vi "AOI_Main.vi"() -> ()   [LabVIEW 2017]
uses:
  <vilib>/userdefined/High Color/IMAQdx.ctl
  <vilib>/vision/driver/IMAQdx.llb/IMAQdx Camera Control Mode.ctl
  <vilib>/Utility/file.llb/Write Delimited Spreadsheet (string).vi
  <vilib>/Utility/file.llb/Read Delimited Spreadsheet (string).vi
  <vilib>/vision/Image Controls.llb/IMAQ Image.ctl
panel:
  out "NG folder array":string[](array[string])
  out "cutting offset\n切割偏移":dbl
  out "damaged\n膠殼破損":dbl
  out "carck\n板裂":dbl
  out "glitch\n毛邊":dbl
  out "number\n數量":dbl
  out "NG code":dbl
  in  "save image\n影像儲存":bool
  in  "output folder\n輸出資料夾":path
  in  "Load setting\n載入參數":bool
  in  "Save setting\n儲存參數":bool
  in  "parameter\n參數":T1={"image imshow (影像繪製)"=FALSE, "side length (mm)\n樣品長度"=0.0, "Main Range (Threshold)\n主輪廓二值化"={"Lower value (上限)"=73.0, "Upper value (下限)"=255.0}, "side velocity threshold\n邊長速度閥值"=0.0, "Sub Range (Threshold)\n次輪廓二值化"={"Lower value (上限)"=73.0, "Upper value (下限)"=255.0}, "close kernel size\n (閉運算核核心大小)"=0.0, "open kernel size\n (開運算核心大小)"=0.0, "side angle offest (threshold)\n邊界角度抑制"=0.0}
  in  "NG_rules( NG規則)":T2
  out "Not DO 2":bool
  out "NG DO 1":bool
  in  "Delay 拍照":u32
  out "img0":T3
  out "Pass DO 0":bool
  out "SOT DI 0":bool
  out "Image\n影像":T3(plugin-control)
  out "TEST.txt Read 2":string[][](array[string])
  out "error Out (no error)":errorcluster
  in  "Exit\n離開":bool
  in  "觸發":bool
  in  "Connect\n連接":bool
  # "人機介面設計尺寸1366*768\n目前檢測硬體可使用解析度"
  # "Design by OPS Automation Innovation Division"
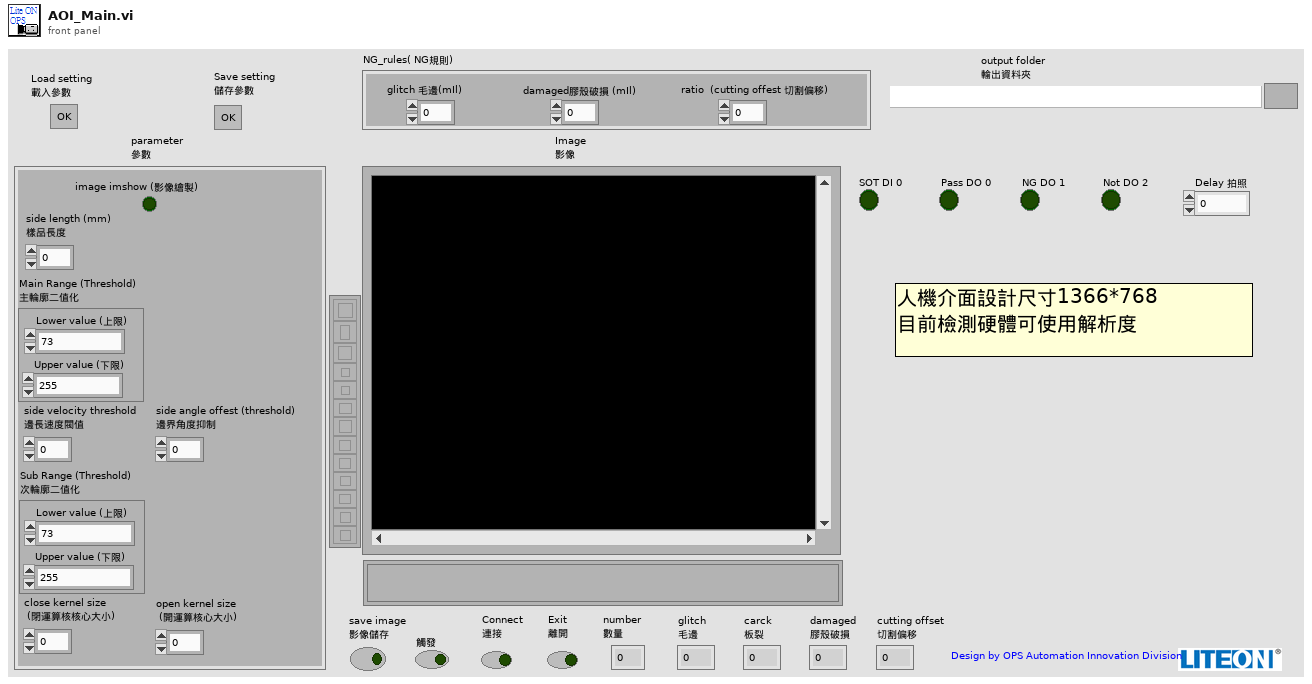
[diagram p1: front panel]
types:
  T1 = cluster{"image imshow (影像繪製)":bool, "side length (mm)\n樣品長度":dbl, "Main Range (Threshold)\n主輪廓二值化":cluster{"Lower value (上限)":sgl, "Upper value (下限)":sgl}, "side velocity threshold\n邊長速度閥值":dbl, "Sub Range (Threshold)\n次輪廓二值化":cluster{"Lower value (上限)":sgl, "Upper value (下限)":sgl}, "close kernel size\n (閉運算核核心大小)":dbl, "open kernel size\n (開運算核心大小)":dbl, "side angle offest (threshold)\n邊界角度抑制":dbl}
  T2 = cluster{"glitch 毛邊(mIl)":dbl, "damaged膠殼破損 (mIl)":dbl, "ratio  (cutting offest 切割偏移)":dbl}
  T3 = typedef "IMAQ Image.ctl" = refnum<image>
  T4 = enum16{"open", "replace", "create", "open or create", "replace or create", "replace or create with confirmation"}
  T5 = typedef "NI_Vision_Acquisition_Software.lvlib/IMAQdx Camera Control Mode.ctl" = enum32{"Controller", "Listener"}
  T6 = typedef "IMAQdx.ctl" = refnum<k21>
  T7 = typedef "Image Type" = u32
  T8 = cluster{"Lower value (上限)":sgl, "Upper value (下限)":sgl}
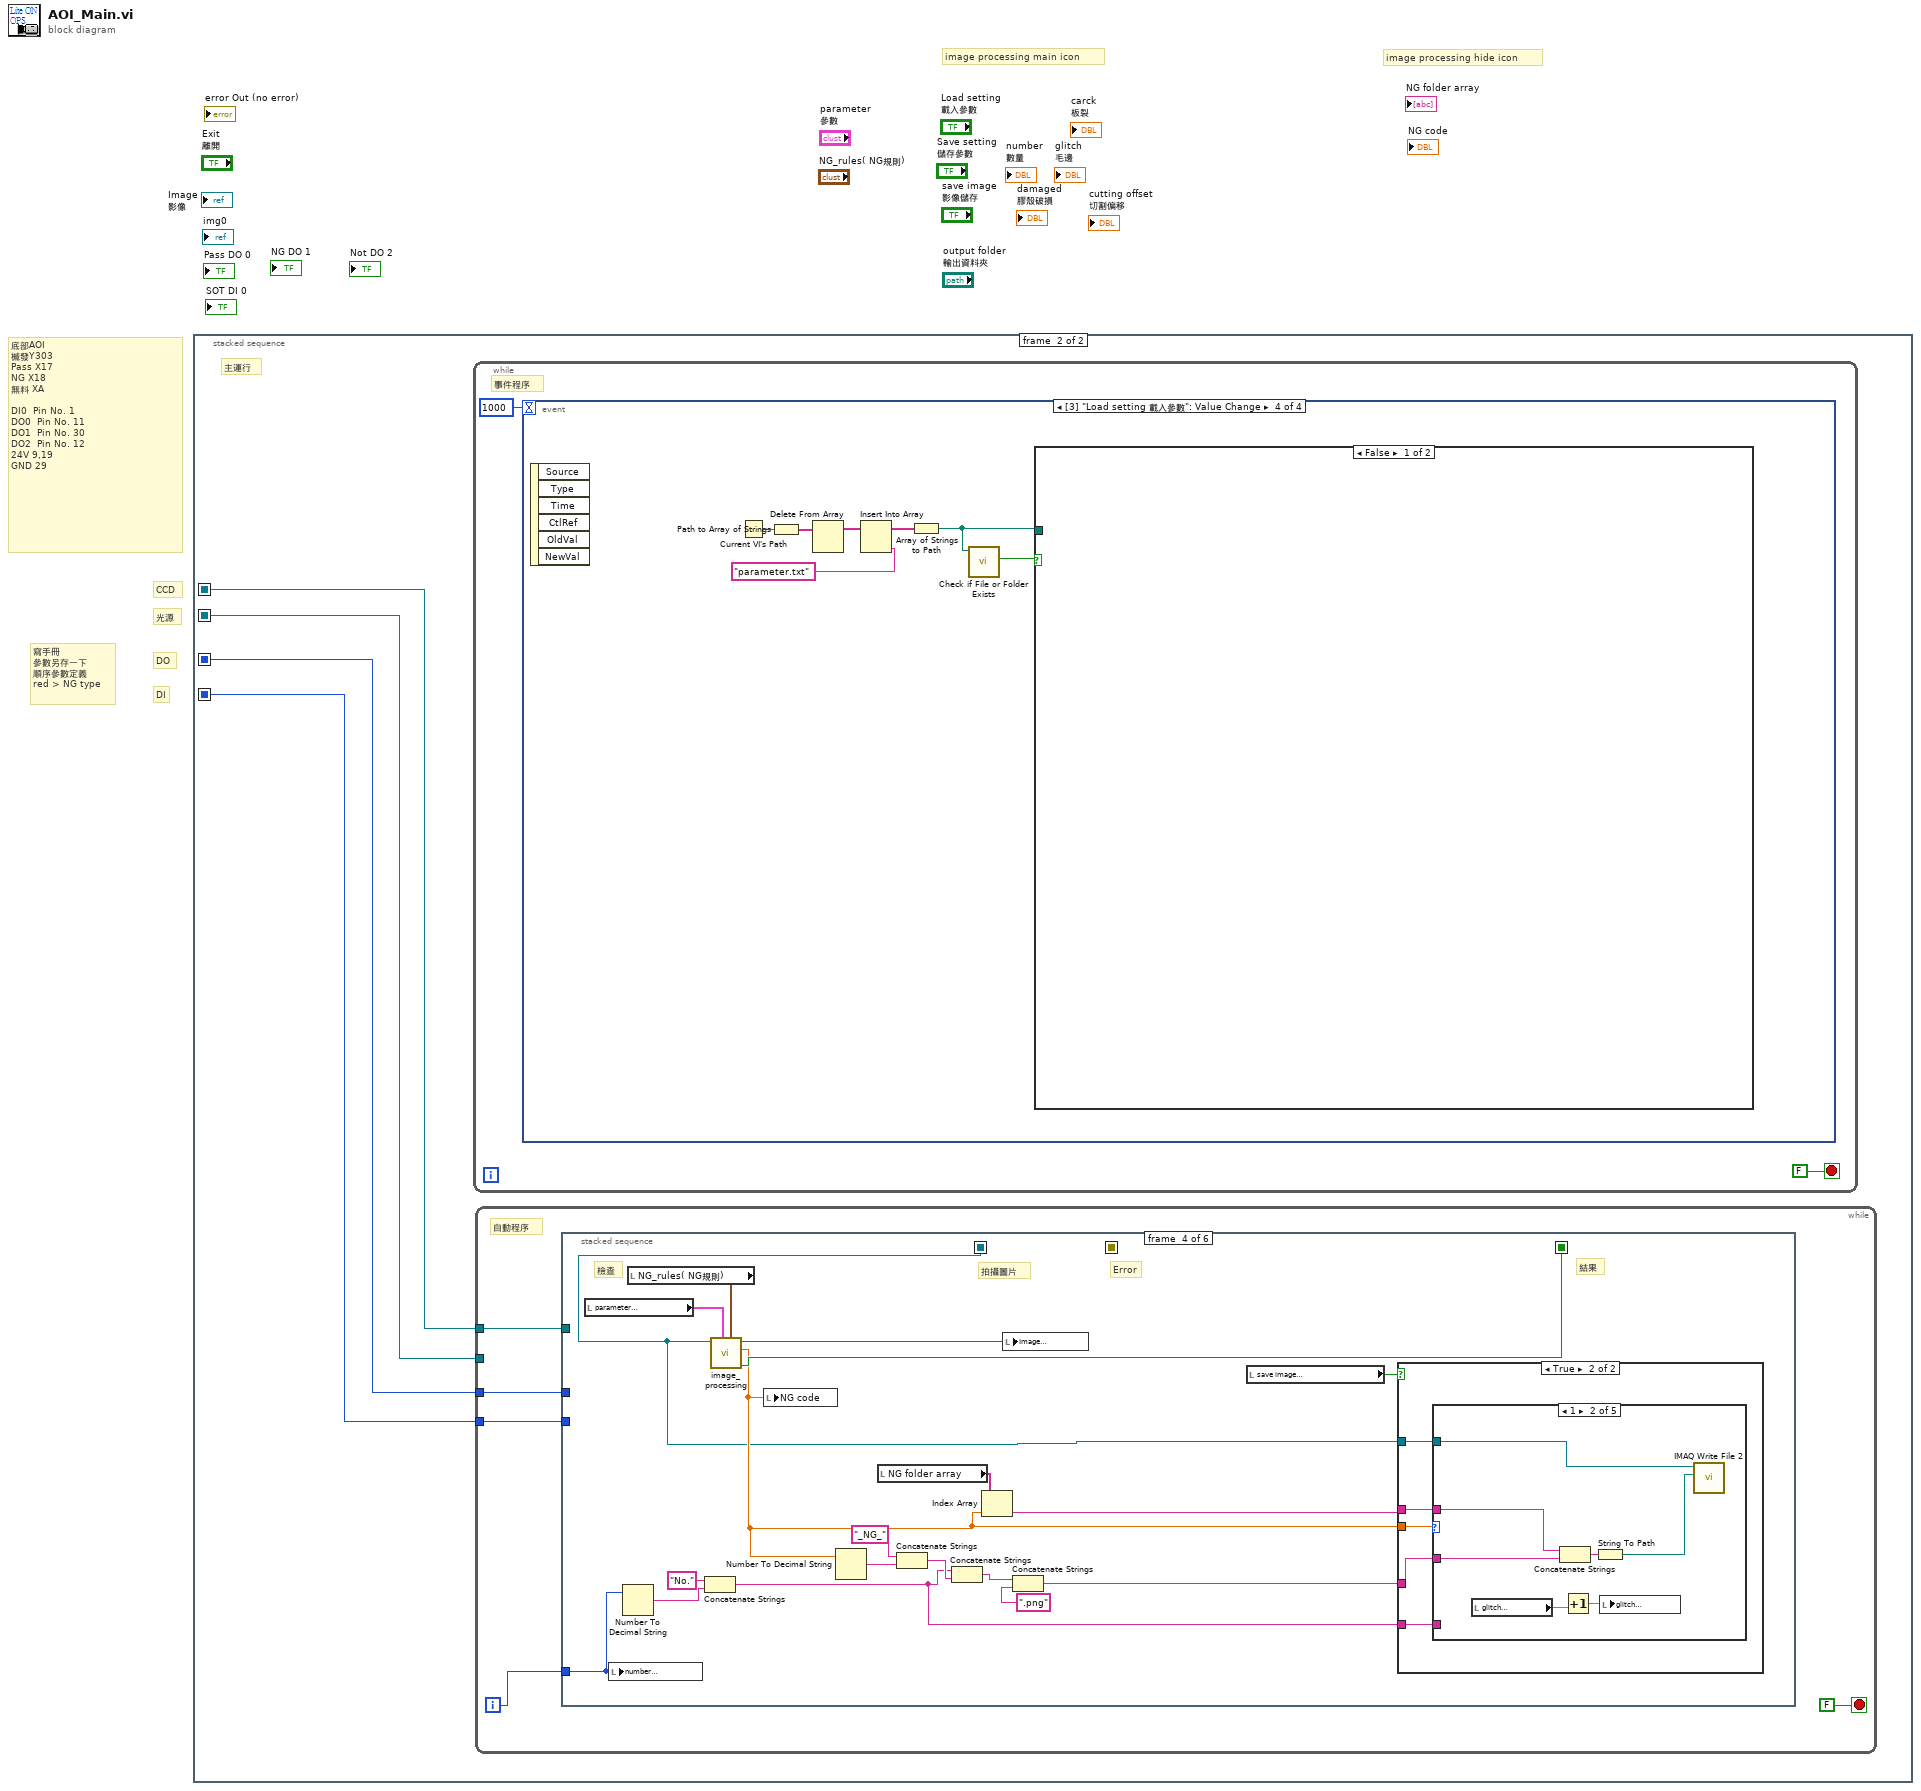
[diagram p0: block diagram]
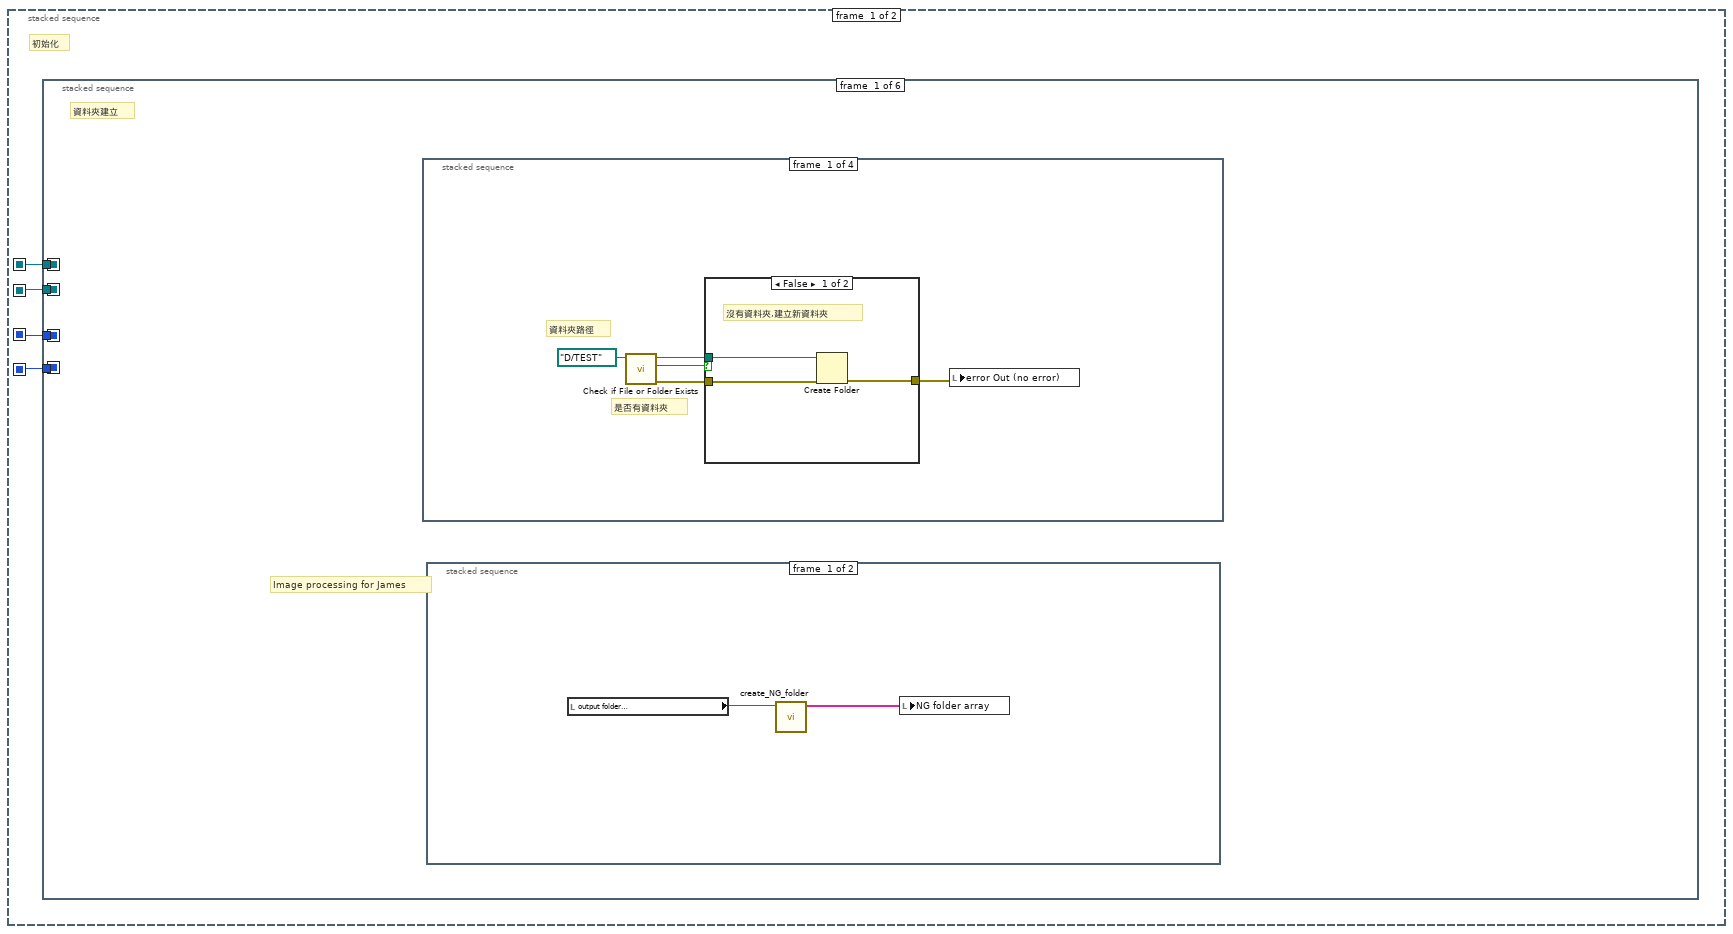
[diagram p2: hidden frame]
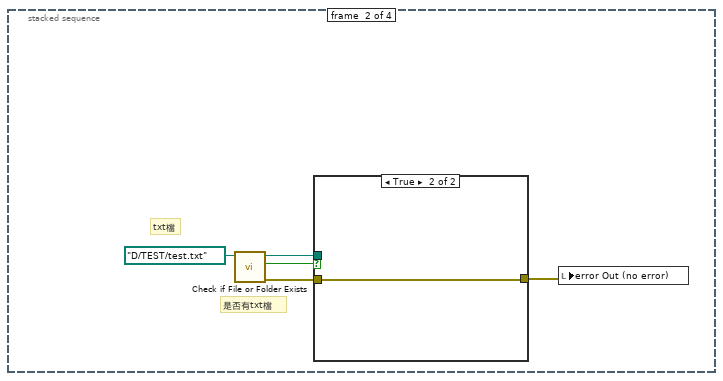
[diagram p5: hidden frame]
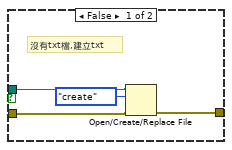
[diagram p6: hidden frame]
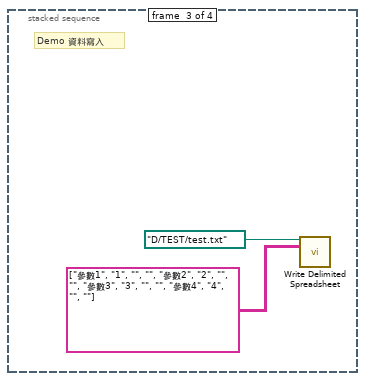
[diagram p7: hidden frame]
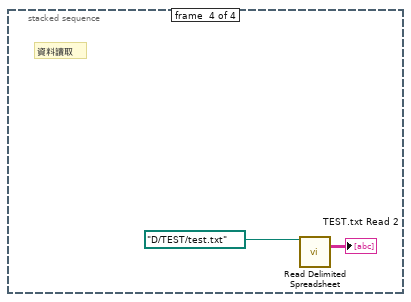
[diagram p8: hidden frame]
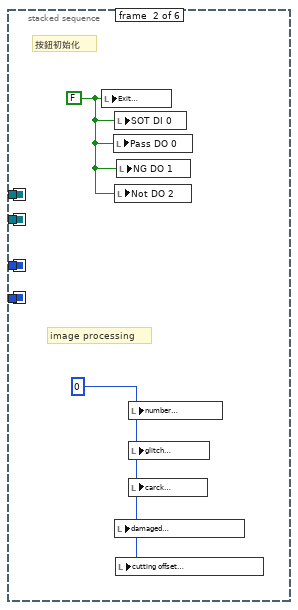
[diagram p9: hidden frame]
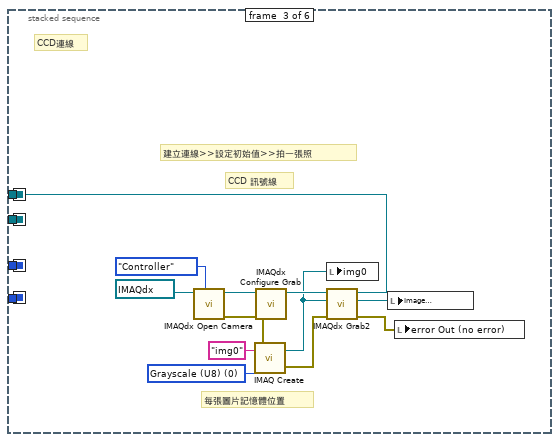
[diagram p10: hidden frame]
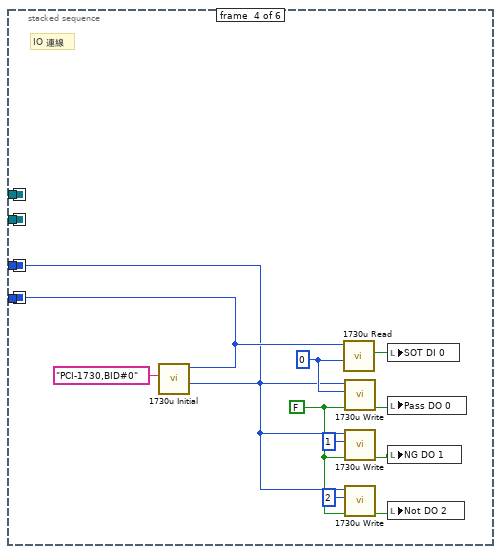
[diagram p11: hidden frame]
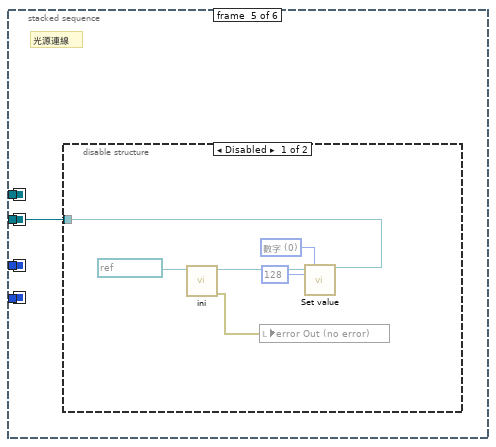
[diagram p12: hidden frame]
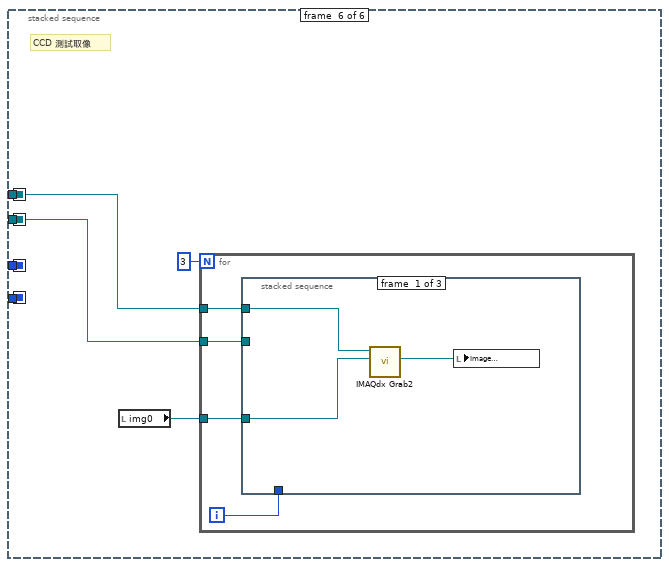
[diagram p14: hidden frame]
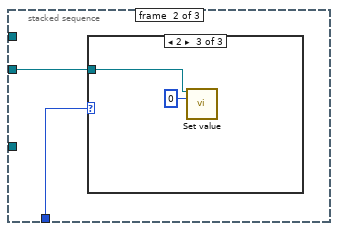
[diagram p15: hidden frame]
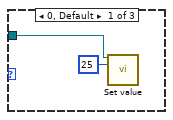
[diagram p16: hidden frame]
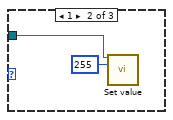
[diagram p17: hidden frame]
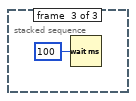
[diagram p18: hidden frame]
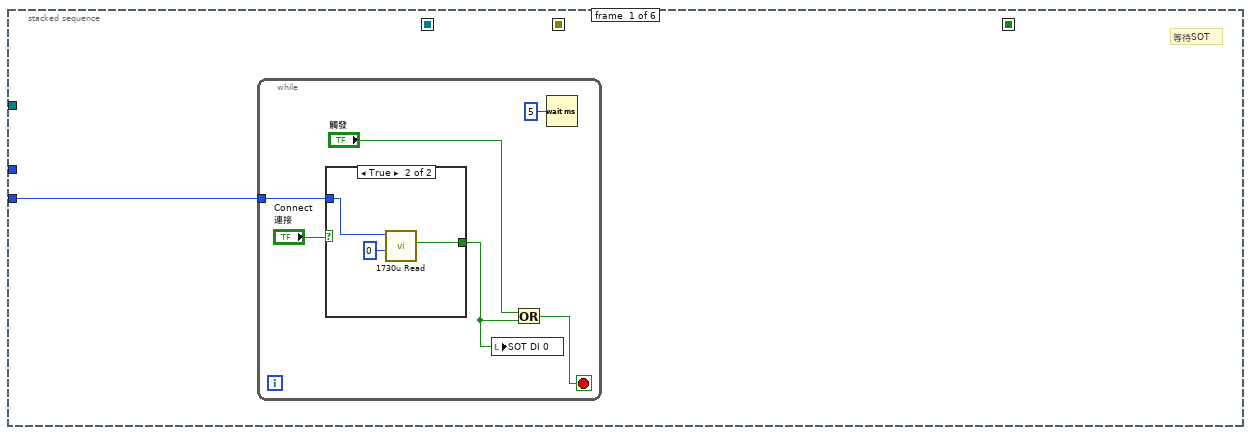
[diagram p19: hidden frame]
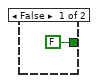
[diagram p20: hidden frame]
diagram:
  # "image processing hide icon"
  # "image processing main icon"
  # "寫手冊\n參數另存一下\n順序參數定義\nred > NG type"
  # "底部AOI\n槭發Y303\nPass X17\nNG X18\n無料 XA\n\nDI0  Pin No. 1\nDO0  Pin No. 11\nDO1  Pin No. 30\nDO2  Pin No. 12\n24V 9,19\nGND 29"
  # "DI"
  # "DO"
  # "光源"
  # "CCD"
  n1 = stacked-sequence {
    seq-local: [w4 _] -> [_ w83]
    seq-local: [w3 _] -> [_ w82]
    seq-local: [w2 _] -> [_ w81]
    seq-local: [w1 _] -> [_ w80]
    frame #0 {
      # "初始化"
      n2 = stacked-sequence {
        seq-local: [_ _ w39 _ _ _] -> [_ _ _ _ _ w63]
        seq-local: [_ _ _ _ w53 _] -> [_ _ _ _ _ w62]
        seq-local: [_ _ _ w50 _ _] -> [_ _ _ _ _ _]
        seq-local: [_ _ _ w48 _ _] -> [_ _ _ _ _ _]
        tunnel: [_ _ w39 _ _ _] -> w4
        tunnel: [_ _ _ _ w53 _] -> w3
        tunnel: [_ _ _ w48 _ _] -> w2
        tunnel: [_ _ _ w50 _ _] -> w1
        frame #0 {
          # "Image processing for James"
          # "資料夾建立"
          n3 = stacked-sequence {
            frame #0 {
              # "是否有資料夾"
              # "資料夾路徑"
              n4 = call <vilib>:"Check if File or Folder Exists.vi"("path"=path "D:/TEST") -> ("error out"=w8:errorcluster, "file or folder exists?"=w10:bool, "dup path"=w9:path)  [unwired: 8 in]
              n5 = case shown="False" w10 {
                tunnel: w9 -> [w14 _]
                tunnel: w8 -> [w13 w15]
                tunnel: [w12 w15] -> w7
                frame False {
                  # "沒有資料夾,建立新資料夾"
                  n6 = Create Folder(path (use dialog)=w14, error in=w13) -> (error out=w12:errorcluster)  [unwired: 1 in, 2 out]
                }
                frame True {
                }
              }
              n7 = local write "error Out (no error)"(w7) -> ()
            }
            frame #1 {
              # "是否有txt檔"
              # "txt檔"
              n8 = call <vilib>:"Check if File or Folder Exists.vi"("path"=path "D:/TEST/test.txt") -> ("error out"=w18:errorcluster, "file or folder exists?"=w20:bool, "dup path"=w19:path)  [unwired: 8 in]
              n9 = case shown="True" w20 {
                tunnel: w19 -> [w24 _]
                tunnel: w18 -> [w23 w25]
                tunnel: [w22 w25] -> w17
                frame False {
                  # "沒有txt檔,建立txt"
                  n10 = Open/Create/Replace File(file path (use dialog)=w24, error in=w23, operation (0:open)=T4."create") -> (error out=w22:errorcluster)  [unwired: 3 in, 2 out]
                }
                frame True {
                }
              }
              n11 = local write "error Out (no error)"(w17) -> ()
            }
            frame #2 {
              # "Demo 資料寫入"
              n12 = call-poly <vilib>:"Write Delimited Spreadsheet.vi"("file path (dialog if empty)"=path "D:/TEST/test.txt" ("path"), "2D data"=string[][] [["參數1", "1", "", ""], ["參數2", "2", "", ""], ["參數3", "3", "", ""], ["參數4", "4", "", ""]]) -> ()  [unwired: 12 in, 2 out]
            }
            frame #3 {
              # "資料讀取"
              n13 = call-poly <vilib>:"Read Delimited Spreadsheet.vi"("file path (dialog if empty)"=path "D:/TEST/test.txt" ("path")) -> ("all rows"=→"TEST.txt Read 2":string[][])  [unwired: 9 in, 5 out]
            }
          }
          n14 = stacked-sequence {
            frame #0 {
              n15 = local read "output folder\n輸出資料夾"() -> (w5:path)
              n16 = call "create_NG_folder.vi"("output folder in"=w5) -> ("NG folder array"=w6:string[])  [unwired: 10 in]
              n17 = local write "NG folder array"(w6) -> ()
            }
            frame #1 {
            }
          }
        }
        frame #1 {
          w30 = 0
          w31 = FALSE ("Exit")
          # "image processing"
          # "按鈕初始化"
          n18 = local write "Exit\n離開"(w31) -> ()
          n19 = local write "Pass DO 0"(w31) -> ()
          n20 = local write "SOT DI 0"(w31) -> ()
          n21 = local write "Not DO 2"(w31) -> ()
          n22 = local write "damaged\n膠殼破損"(w30) -> ()
          n23 = local write "cutting offset\n切割偏移"(w30) -> ()
          n24 = local write "NG DO 1"(w31) -> ()
          n25 = local write "number\n數量"(w30) -> ()
          n26 = local write "glitch\n毛邊"(w30) -> ()
          n27 = local write "carck\n板裂"(w30) -> ()
        }
        frame #2 {
          w35 = T7 0 items=["Grayscale (U8)", "Grayscale (I16)", "Grayscale (SGL)", "Complex (CSG)", "RGB (U32)", "HSL (U32)", "RGB (U64)", "Grayscale (U16)"] ("Image Type")
          # "每張圖片記憶體位置"
          # "建立連線>>設定初始值>>拍一張照"
          # "CCD 訊號線"
          # "CCD連線"
          n28 = call <vilib>:"IMAQdx Open Camera.vi"("Camera Control Mode"=IMAQdx_Camera_Control_Mode."Controller", "Session In"=T6 "cam0") -> ("error out"=w42:errorcluster, "Session Out"=w43:T6)  [unwired: 8 in]
          n29 = call <vilib>:"IMAQdx Configure Grab.vi"("error in"=w42, "Session In"=w43) -> ("error out"=w38:errorcluster, "Session Out"=w40:T6)  [unwired: 8 in]
          n30 = call "IMAQ Create"("Image Name"="img0", "Image Type"=w35, "error in (no error)"=w38) -> ("New Image"=w32:T3, "error out"=w37:errorcluster)  [unwired: 2 in]
          n31 = local write "img0"(w32) -> ()
          n32 = call <vilib>:"IMAQdx Grab2.vi"("error in"=w37, "Image In"=w32, "Session In"=w40) -> ("error out"=w33:errorcluster, "Image Out"=w34:T3, "Session Out"=w39:T6)  [unwired: 5 in, 1 out]
          n33 = local write "Image\n影像"(w34) -> ()
          n34 = local write "error Out (no error)"(w33) -> ()
        }
        frame #3 {
          w45 = FALSE ("data")
          w51 = 0 ("portBit")
          # "IO 連線"
          n35 = call <userlib>:"1730u Initial.vi"("physical channels"="PCI-1730,BID#0") -> ("task DO 0~7"=w48:i32, "task DI 0~7"=w50:i32)  [unwired: 6 in, 3 out]
          n36 = call <userlib>:"1730u Read.vi"("portBit"=w51, "DI task in"=w50) -> ("data"=w49:bool)  [unwired: 8 in, 1 out]
          n37 = call <userlib>:"1730u Write.vi"("data"=w45, "portBit"=w51, "DO task in"=w48) -> ()  [unwired: 8 in, 1 out]
          n38 = call <userlib>:"1730u Write.vi"("data"=w45, "portBit"=1, "DO task in"=w48) -> ()  [unwired: 8 in, 1 out]
          n39 = call <userlib>:"1730u Write.vi"("data"=w45, "portBit"=2, "DO task in"=w48) -> ()  [unwired: 8 in, 1 out]
          n40 = local write "SOT DI 0"(w49) -> ()
          n41 = local write "Pass DO 0"(w45) -> ()
          n42 = local write "NG DO 1"(w45) -> ()
          n43 = local write "Not DO 2"(w45) -> ()
        }
        frame #4 {
          # "光源連線"
          n44 = disable-structure shown="Disabled" {
            disable-tunnel: [w56 _] -> w53
            frame Disabled {
              w57 = u16 0 items=["數字", "閃頻"] ("CST Ctr mode")
              n45 = call <userlib>:"ini.vi"("VISA resource name"=refnum<visa-resource-name> "COM3") -> ("error out"=w55:errorcluster, "VISA resource name out"=w58:refnum<visa-resource-name>)  [unwired: 9 in]
              n46 = local write "error Out (no error)"(w55) -> ()
              n47 = call <userlib>:"Set value.vi"("VISA resource name"=w58, "CST Ctr mode"=w57, "CH1"=i16 128) -> ("VISA resource name out"=w56:refnum<visa-resource-name>)  [unwired: 12 in]
            }
            frame Enabled {
            }
          }
        }
        frame #5 {
          # "CCD 測試取像"
          n48 = local read "img0"() -> (w60:T3)
          n49 = for {
            N: 3 -> [_]
            tunnel: w63 -> [w67]
            tunnel: w62 -> [w65]
            tunnel: w60 -> [w66]
            i -> [w64]
            n50 = stacked-sequence {
              tunnel: w67 -> [w70 _ _]
              tunnel: w66 -> [w69 _ _]
              tunnel: w65 -> [_ w71 _]
              tunnel: w64 -> [_ w72 _]
              frame #0 {
                n51 = call <vilib>:"IMAQdx Grab2.vi"("Image In"=w69, "Session In"=w70) -> ("Image Out"=w68:T3)  [unwired: 6 in, 3 out]
                n52 = local write "Image\n影像"(w68) -> ()
              }
              frame #1 {
                n53 = case shown="2" w72 {
                  tunnel: w71 -> [w74 w76 w78]
                  frame 0, Default {
                    n54 = call <userlib>:"Set value.vi"("VISA resource name"=w74, "CH1"=i16 25) -> ()  [unwired: 13 in, 1 out]
                  }
                  frame 1 {
                    n55 = call <userlib>:"Set value.vi"("VISA resource name"=w76, "CH1"=i16 255) -> ()  [unwired: 13 in, 1 out]
                  }
                  frame 2 {
                    n56 = call <userlib>:"Set value.vi"("VISA resource name"=w78, "CH1"=i16 0) -> ()  [unwired: 13 in, 1 out]
                  }
                }
              }
              frame #2 {
                n57 = Wait (ms)(milliseconds to wait=u32 100) -> ()  [unwired: 1 out]
              }
            }
          }
        }
      }
    }
    frame #1 {
      # "主運行"
      n58 = while {
        stop <- FALSE stop-if-true
        # "事件程序"
        n59 = event shown="[3] \"Load setting 載入參數\": Value Change" {
          selector: _ -> [_ _ _ _]
          dyn-events: _ -> [_ _ _ _]
          timeout: 1000 -> [_ _ _ _]
          event Timeout {
            n60 = event-data() -> ()  [unwired: 1 in, 3 out]
          }
          event "Exit\n離開": Value Change {
            n61 = event-data() -> ()  [unwired: 1 in, 6 out]
            n62 = stacked-sequence {
              frame #0 {
                # "初始化設備"
              }
              frame #1 {
                # "關閉 LabVIEW"
                n63 = Quit LabVIEW(quit? (T)=TRUE) -> ()
              }
            }
          }
          event "Save setting\n儲存參數": Value Change {
            n64 = event-data() -> ()  [unwired: 1 in, 6 out]
            n65 = Current VI's Path() -> (path=w203:path)
            n66 = Path to Array of Strings(0:w203) -> (2:w204:string[])  [unwired: 1 out]
            n67 = Delete From Array(array=w204) -> (array with subset deleted=w205:string[])  [unwired: 2 in, 1 out]
            n68 = Insert Into Array(array=w205, new element="parameter.txt" ("string")) -> (w206:string[])  [unwired: 1 in]
            n69 = Array of Strings to Path(0:w206) -> (2:w202:path)  [unwired: 1 in]
            n70 = call <vilib>:"Check if File or Folder Exists.vi"("path"=w202) -> ("file or folder exists?"=w201:bool)  [unwired: 8 in, 2 out]
            n71 = stacked-sequence {
              seq-local: [_ w210 _ _] -> [_ _ w229 _]
              tunnel: w202 -> [w208 w211 _ _]
              tunnel: w201 -> [w207 _ _ _]
              frame #0 {
                n72 = case shown="False" w207 {
                  tunnel: w208 -> [_ w209]
                  frame False {
                  }
                  frame True {
                    n73 = Delete(path (use dialog)=w209) -> ()  [unwired: 4 in, 3 out]
                  }
                }
              }
              frame #1 {
                n74 = local read "NG_rules( NG規則)"() -> (w218:T2)
                n75 = local read "parameter\n參數"() -> (w228:T1)
                n76 = Unbundle(w228) -> ("side length (mm)\n樣品長度"=w225:dbl, "Main Range (Threshold)\n主輪廓二值化"=w226:T8, "side velocity threshold\n邊長速度閥值"=w222:dbl, "Sub Range (Threshold)\n次輪廓二值化"=w227:T8, "close kernel size\n (閉運算核核心大小)"=w219:dbl, "open kernel size\n (開運算核心大小)"=w213:dbl, "side angle offest (threshold)\n邊界角度抑制"=w212:dbl)  [unwired: 1 out]
                n77 = Cluster To Array(cluster=w218) -> (array=w217:dbl[])
                n78 = Unbundle(w226) -> ("Lower value (上限)"=w224:sgl, "Upper value (下限)"=w223:sgl)
                n79 = Unbundle(w227) -> ("Lower value (上限)"=w221:sgl, "Upper value (下限)"=w220:sgl)
                n80 = call "np_astype_str.vi"("NG_rules"=w217) -> ("Array"=w216:string[])  [unwired: 10 in]
                n81 = Build Array(w225, w224, w223, w222, w221, w220, w219, w213, w212) -> (w215:dbl[])
                n82 = call "np_astype_str.vi"("NG_rules"=w215) -> ("Array"=w214:string[])  [unwired: 10 in]
                n83 = Build Array(w216, w214) -> (w210:string[][])
                n84 = call-poly <vilib>:"Write Delimited Spreadsheet.vi"("file path (dialog if empty)"=w211, "2D data"=w210) -> ()  [unwired: 12 in, 2 out]
              }
              frame #2 {
                n85 = call "re_create_folder.vi"("output folder in"=path "C:/userss") -> ("output folder out"=w235:path)  [unwired: 10 in]
                n86 = Path to Array of Strings(0:w235) -> (2:w238:string[])  [unwired: 1 out]
                n87 = Delete From Array(array=w238) -> (array with subset deleted=w237:string[])  [unwired: 2 in, 1 out]
                n88 = Insert Into Array(array=w237, new element="userss" ("string")) -> (w234:string[])  [unwired: 1 in]
                n89 = Insert Into Array(array=w234, new element="parameter.txt" ("string")) -> (w233:string[])  [unwired: 1 in]
                n90 = Array of Strings to Path(0:w233) -> (2:w230:path)  [unwired: 1 in]
                n91 = call-poly <vilib>:"Write Delimited Spreadsheet.vi"("file path (dialog if empty)"=w230, "2D data"=w229, "append to file? (new file:F)"=w231) -> ("1D data"=w231:string[])  [unwired: 10 in, 2 out]
              }
              frame #3 {
                n92 = One Button Dialog(message="Save success!") -> ()  [unwired: 1 in, 1 out]
              }
            }
          }
          event "Load setting\n載入參數": Value Change {
            n93 = event-data() -> ()  [unwired: 1 in, 6 out]
            n94 = Current VI's Path() -> (path=w244:path)
            n95 = Path to Array of Strings(0:w244) -> (2:w245:string[])  [unwired: 1 out]
            n96 = Delete From Array(array=w245) -> (array with subset deleted=w246:string[])  [unwired: 2 in, 1 out]
            n97 = Insert Into Array(array=w246, new element="parameter.txt" ("string")) -> (w247:string[])  [unwired: 1 in]
            n98 = Array of Strings to Path(0:w247) -> (2:w243:path)  [unwired: 1 in]
            n99 = call <vilib>:"Check if File or Folder Exists.vi"("path"=w243) -> ("file or folder exists?"=w242:bool)  [unwired: 8 in, 2 out]
            n100 = case shown="False" w242 {
              tunnel: w243 -> [_ w249]
              frame False {
              }
              frame True {
                n101 = call-poly <vilib>:"Read Delimited Spreadsheet.vi"("file path (dialog if empty)"=w249) -> ("all rows"=w248:string[][])  [unwired: 9 in, 5 out]
                n102 = stacked-sequence {
                  tunnel: w248 -> [w258 w297 _]
                  frame #0 {
                    n103 = Index Array(array=w258, index (row)=1) -> (element=w272:string[])  [unwired: 1 in]
                    n104 = Index Array(array=w258, index (row)=1) -> (element=w259:string[])  [unwired: 1 in]
                    n105 = Index Array(array=w258, index (row)=1) -> (element=w265:string[])  [unwired: 1 in]
                    n106 = Index Array(array=w258, index (row)=1) -> (element=w264:string[])  [unwired: 1 in]
                    n107 = Index Array(array=w272, index=2 ("index (row)")) -> (element=w253:string)
                    n108 = Index Array(array=w259, index=1 ("index (row)")) -> (element=w252:string)
                    n109 = Index Array(array=w265, index=4 ("index (row)")) -> (element=w251:string)
                    n110 = Index Array(array=w264, index=5 ("index (row)")) -> (element=w250:string)
                    n111 = Scan From String(input string=w252) -> (output 1=w257:dbl)  [unwired: 4 in, 3 out]
                    n112 = Scan From String(input string=w253) -> (output 1=w256:dbl)  [unwired: 4 in, 3 out]
                    n113 = Scan From String(input string=w251) -> (output 1=w255:dbl)  [unwired: 4 in, 3 out]
                    n114 = Scan From String(input string=w250) -> (output 1=w254:dbl)  [unwired: 4 in, 3 out]
                    n115 = local read "parameter\n參數"() -> (w270:T1)
                    n116 = Bundle By Name(cluster=w270, "Main Range (Threshold)\n主輪廓二值化.Lower value (上限)"=w257, "Main Range (Threshold)\n主輪廓二值化.Upper value (下限)"=w256, "Sub Range (Threshold)\n次輪廓二值化.Lower value (上限)"=w255, "Sub Range (Threshold)\n次輪廓二值化.Upper value (下限)"=w254) -> (w269:T1)
                    n117 = local write "parameter\n參數"(w269) -> ()
                  }
                  frame #1 {
                    n118 = Index Array(array=w297, index (row)=1) -> (element=w273:string[])  [unwired: 1 in]
                    n119 = Index Array(array=w297, index (row)=0) -> (element=w299:string[])  [unwired: 1 in]
                    n120 = Index Array(array=w273, index=8 ("index (row)")) -> (element=w276:string)
                    n121 = Index Array(array=w273, index=7 ("index (row)")) -> (element=w283:string)
                    n122 = Index Array(array=w273, index=6 ("index (row)")) -> (element=w284:string)
                    n123 = Index Array(array=w273, index=3 ("index (row)")) -> (element=w285:string)
                    n124 = Index Array(array=w299, index=1 ("index (row)")) -> (element=w288:string)
                    n125 = Index Array(array=w273, index=0 ("index (row)")) -> (element=w286:string)
                    n126 = Index Array(array=w299, index=0 ("index (row)")) -> (element=w289:string)
                    n127 = Index Array(array=w299, index=2 ("index (row)")) -> (element=w287:string)
                    n128 = Scan From String(input string=w276) -> (output 1=w274:dbl)  [unwired: 4 in, 3 out]
                    n129 = Scan From String(input string=w287) -> (output 1=w281:dbl)  [unwired: 4 in, 3 out]
                    n130 = Scan From String(input string=w283) -> (output 1=w277:dbl)  [unwired: 4 in, 3 out]
                    n131 = Scan From String(input string=w289) -> (output 1=w290:dbl)  [unwired: 4 in, 3 out]
                    n132 = Scan From String(input string=w288) -> (output 1=w282:dbl)  [unwired: 4 in, 3 out]
                    n133 = Scan From String(input string=w286) -> (output 1=w280:dbl)  [unwired: 4 in, 3 out]
                    n134 = Scan From String(input string=w285) -> (output 1=w279:dbl)  [unwired: 4 in, 3 out]
                    n135 = Scan From String(input string=w284) -> (output 1=w278:dbl)  [unwired: 4 in, 3 out]
                    n136 = local read "NG_rules( NG規則)"() -> (w300:T2)
                    n137 = Bundle By Name(cluster=w300, "glitch 毛邊(mIl)"=w290, "damaged膠殼破損 (mIl)"=w282, "ratio  (cutting offest 切割偏移)"=w281) -> (w303:T2)
                    n138 = local read "parameter\n參數"() -> (w291:T1)
                    n139 = Bundle By Name(cluster=w291, "side length (mm)\n樣品長度"=w280, "side velocity threshold\n邊長速度閥值"=w279, "close kernel size\n (閉運算核核心大小)"=w278, "open kernel size\n (開運算核心大小)"=w277, "side angle offest (threshold)\n邊界角度抑制"=w274) -> (w295:T1)
                    n140 = local write "NG_rules( NG規則)"(w303) -> ()
                    n141 = local write "parameter\n參數"(w295) -> ()
                  }
                  frame #2 {
                    n142 = One Button Dialog(message="Save success!") -> ()  [unwired: 1 in, 1 out]
                  }
                }
              }
            }
          }
        }
      }
      n143 = while {
        tunnel: w83 -> [w85]
        tunnel: w82 -> [_]
        tunnel: w81 -> [w86]
        tunnel: w80 -> [w87]
        i -> [w84]
        stop <- FALSE stop-if-true
        # "自動程序"
        n144 = stacked-sequence {
          seq-local: [_ _ w109 _ _ _] -> [_ _ _ w117 _ _]
          seq-local: [_ _ w107 _ _ _] -> [_ _ _ _ _ _]
          seq-local: [_ _ _ w133 _ _] -> [_ _ _ _ w179 _]
          tunnel: w87 -> [w89 _ _ _ _ w196]
          tunnel: w86 -> [_ w106 _ _ w185 _]
          tunnel: w85 -> [_ _ w110 _ _ _]
          tunnel: w84 -> [_ _ _ w125 _ _]
          frame #0 {
            # "等待SOT"
            n145 = while {
              tunnel: w89 -> [w91]
              stop <- w95 stop-if-true
              n146 = case shown="True" "Connect\n連接" {
                tunnel: w91 -> [_ w99]
                tunnel: [FALSE ("data") w97] -> w90
                frame False {
                }
                frame True {
                  n147 = call <userlib>:"1730u Read.vi"("portBit"=0, "DI task in"=w99) -> ("data"=w97:bool)  [unwired: 8 in, 1 out]
                }
              }
              n148 = local write "SOT DI 0"(w90) -> ()
              n149 = Or(x="觸發", y=w90) -> (x .or. y?=w95:bool)
              n150 = Wait (ms)(milliseconds to wait=u32 5) -> ()  [unwired: 1 out]
            }
          }
          frame #1 {
            w100 = FALSE ("data")
            # "EOT 切換\nArray整理"
            n151 = local write "Pass DO 0"(w100) -> ()
            n152 = call <userlib>:"1730u Write.vi"("data"=w100, "portBit"=0, "DO task in"=w106) -> ("DO task out"=w103:i32)  [unwired: 8 in]
            n153 = local write "NG DO 1"(w100) -> ()
            n154 = call <userlib>:"1730u Write.vi"("data"=w100, "portBit"=1, "DO task in"=w103) -> ("DO task out"=w102:i32)  [unwired: 8 in]
            n155 = local write "Not DO 2"(w100) -> ()
            n156 = call <userlib>:"1730u Write.vi"("data"=w100, "portBit"=2, "DO task in"=w102) -> ()  [unwired: 8 in, 1 out]
          }
          frame #2 {
            # "取像"
            n157 = flat-sequence {
              tunnel: w110 -> [w112]
              tunnel: [w112] -> w108
              tunnel: [w114] -> w109
              tunnel: w108 -> [w116]
              tunnel: [w113] -> w107
              frame #0 {
                n158 = Wait (ms)(milliseconds to wait="Delay 拍照") -> ()  [unwired: 1 out]
              }
              frame #1 {
                n159 = local read "img0"() -> (w115:T3)
                n160 = call <vilib>:"IMAQdx Grab2.vi"("Image In"=w115, "Session In"=w116) -> ("error out"=w113:errorcluster, "Image Out"=w114:T3)  [unwired: 6 in, 2 out]
                n161 = local write "Image\n影像"(w114) -> ()
              }
            }
          }
          frame #3 {
            # "結果"
            # "Error"
            # "拍攝圖片"
            # "檢查"
            n162 = local read "parameter\n參數"() -> (w135:T1)
            n163 = local write "number\n數量"(w125) -> ()
            n164 = Number To Decimal String(number=w125) -> (decimal integer string=w128:string)  [unwired: 1 in]
            n165 = local read "NG_rules( NG規則)"() -> (w134:T2)
            n166 = Concatenate Strings("No." ("string"), w128) -> (w123:string)
            n167 = call "image_processing.vi"("NG_rules"=w134, "parameter"=w135, "image"=w117) -> ("PASS"=w133:bool, "NG code"=w121:dbl, "display image"=w118:T3)  [unwired: 5 in, 1 out]
            n168 = local write "NG code"(w121) -> ()
            n169 = Number To Decimal String(number=w121) -> (decimal integer string=w131:string)  [unwired: 1 in]
            n170 = local read "NG folder array"() -> (w124:string[])
            n171 = Concatenate Strings("_NG_" ("string"), w131) -> (w126:string)
            n172 = Concatenate Strings(w123, w126) -> (w127:string)
            n173 = Index Array(array=w124, index=w121) -> (element=w120:string)
            n174 = local write "Image\n影像"(w118) -> ()
            n175 = Concatenate Strings(w127, ".png" ("string")) -> (w122:string)
            n176 = local read "save image\n影像儲存"() -> (w119:bool)
            n177 = case shown="True" w119 {
              tunnel: w117 -> [_ w140]
              tunnel: w122 -> [_ w139]
              tunnel: w121 -> [_ w136]
              tunnel: w120 -> [_ w138]
              tunnel: w123 -> [_ w137]
              frame False {
              }
              frame True {
                n178 = case shown="1" w136 {
                  tunnel: w140 -> [w145 w154 w158 w166 w173]
                  tunnel: w139 -> [_ w151 w159 w165 w172]
                  tunnel: w138 -> [w144 w148 w155 w162 w169]
                  tunnel: w137 -> [w143 _ _ _ _]
                  frame 0, Default {
                    n179 = Concatenate Strings(w143, ".bmp" ("string")) -> (w141:string)
                    n180 = Concatenate Strings(w144, w141) -> (w146:string)
                    n181 = String To Path(string=w146) -> (path=w147:path)
                    n182 = call-poly "IMAQ Write File 2"("File Path"=w147, "Image"=w145) -> ()  [unwired: 8 in, 2 out]
                  }
                  frame 1 {
                    n183 = local read "glitch\n毛邊"() -> (w150:dbl)
                    n184 = Concatenate Strings(w148, w151) -> (w152:string)
                    n185 = Increment(x=w150) -> (x+1=w149:dbl)
                    n186 = String To Path(string=w152) -> (path=w153:path)
                    n187 = local write "glitch\n毛邊"(w149) -> ()
                    n188 = call-poly "IMAQ Write File 2"("File Path"=w153, "Image"=w154) -> ()  [unwired: 8 in, 2 out]
                  }
                  frame 2 {
                    n189 = local read "carck\n板裂"() -> (w157:dbl)
                    n190 = Concatenate Strings(w155, w159) -> (w160:string)
                    n191 = Increment(x=w157) -> (x+1=w156:dbl)
                    n192 = String To Path(string=w160) -> (path=w161:path)
                    n193 = local write "carck\n板裂"(w156) -> ()
                    n194 = call-poly "IMAQ Write File 2"("File Path"=w161, "Image"=w158) -> ()  [unwired: 8 in, 2 out]
                  }
                  frame 3 {
                    n195 = local read "damaged\n膠殼破損"() -> (w164:dbl)
                    n196 = Concatenate Strings(w162, w165) -> (w167:string)
                    n197 = Increment(x=w164) -> (x+1=w163:dbl)
                    n198 = String To Path(string=w167) -> (path=w168:path)
                    n199 = local write "damaged\n膠殼破損"(w163) -> ()
                    n200 = call-poly "IMAQ Write File 2"("File Path"=w168, "Image"=w166) -> ()  [unwired: 8 in, 2 out]
                  }
                  frame 4 {
                    n201 = local read "cutting offset\n切割偏移"() -> (w171:dbl)
                    n202 = Concatenate Strings(w169, w172) -> (w174:string)
                    n203 = Increment(x=w171) -> (x+1=w170:dbl)
                    n204 = local write "cutting offset\n切割偏移"(w170) -> ()
                    n205 = String To Path(string=w174) -> (path=w175:path)
                    n206 = call-poly "IMAQ Write File 2"("File Path"=w175, "Image"=w173) -> ()  [unwired: 8 in, 2 out]
                  }
                }
              }
            }
          }
          frame #4 {
            w178 = FALSE ("data")
            # "結果輸出"
            n207 = case shown="False" w179 {
              tunnel: [TRUE TRUE] -> w176
              tunnel: [TRUE FALSE] -> w177
              frame False {
                # "NG"
              }
              frame True {
                # "PASS"
              }
            }
            n208 = local write "Pass DO 0"(w176) -> ()
            n209 = call <userlib>:"1730u Write.vi"("data"=w176, "portBit"=0, "DO task in"=w185) -> ("DO task out"=w182:i32)  [unwired: 8 in]
            n210 = local write "NG DO 1"(w177) -> ()
            n211 = call <userlib>:"1730u Write.vi"("data"=w177, "portBit"=1, "DO task in"=w182) -> ("DO task out"=w181:i32)  [unwired: 8 in]
            n212 = call <userlib>:"1730u Write.vi"("data"=w178, "portBit"=2, "DO task in"=w181) -> ()  [unwired: 8 in, 1 out]
            n213 = local write "Not DO 2"(w178) -> ()
          }
          frame #5 {
            # "EOT 結束\n資料整理"
            n214 = Bundle("task DI 0~7"=w196, 0, FALSE) -> (w192:cluster{"task DI 0~7":i32, i32, bool})  [unwired: 1 in]
            n215 = call <userlib>:"Check DI State 1730u.vi"("Time Out"=u32 3000, "Scan time"=u32 2, "Mode"=enum16{"Check One DI", "Check Two DI"}."Check One DI", "1 DI Mode"=w192) -> ()  [unwired: 7 in, 1 out]
          }
        }
      }
    }
  }
